vi "Aircraft 7 GPS Values .vi"(7 "Method":enum16{"Get", "Set"}(ring), 11 "Aircraft GPS Data In":T1) -> (3 "Aircraft GPS Data Out":T1)   [LabVIEW 2014]
uses:
  Controls/Aircraft GPS Data.ctl
  Controls/GPS Fix Type.ctl
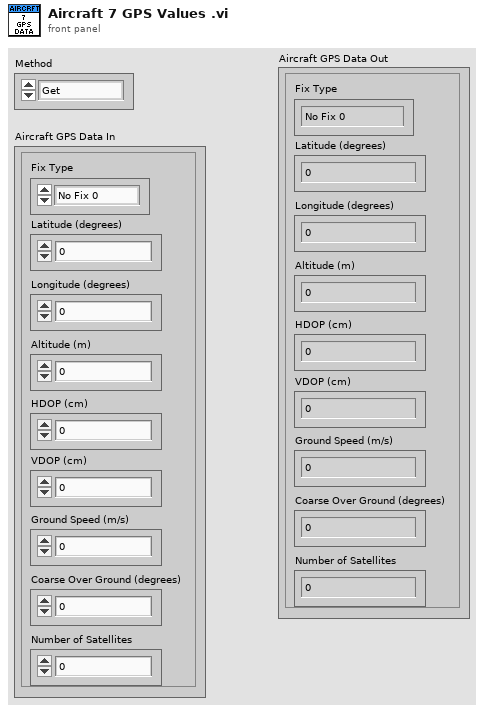
[diagram p1: front panel]
types:
  T1 = typedef "Aircraft GPS Data.ctl" = cluster{"Latitude (degrees)":dbl, "Longitude (degrees)":dbl, "Altitude (m)":dbl, "Fix Type":T2, "HDOP (cm)":u16, "VDOP (cm)":u16, "Ground Speed (m/s)":dbl, "Coarse Over Ground (degrees)":u16, "Number of Satellites":u8}
  T2 = typedef "GPS Fix Type.ctl" = enum16{"No Fix 0", "No Fix 1", "2D Fix", "3D Fix", "DGPS", "RTK"}
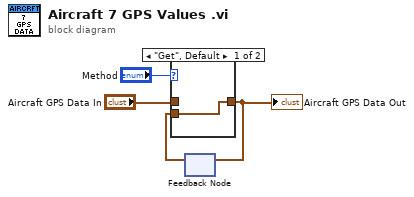
[diagram p0: block diagram]
diagram:
  n1 = feedback #1() -> (w3:T1)  [unwired: 1 in]
  n2 = case shown="\"Get\", Default" "Method" {
    tunnel: "Aircraft GPS Data In" -> [_ w6]
    tunnel: [w5 w6] -> w2
    tunnel: w3 -> [w5 _]
    frame "Get", Default {
    }
    frame "Set" {
    }
  }
  "Aircraft GPS Data Out" <- w2
  n3 = feedback-in #1(w2) -> ()
